vi "Scan time Input.vi"(11 "In":u32=30) -> (3 "out":u32)   [LabVIEW 2011]
doc: "ID=0x6001"
uses:
  <vilib>/Utility/miscctls.llb/LVSelectionTypeDef.ctl
panel:
  in  "cancel":bool
  in  "ok":bool
  in  "Scan Time":u32=10 caption="请输入数值:" min=1 max=10000 step=1
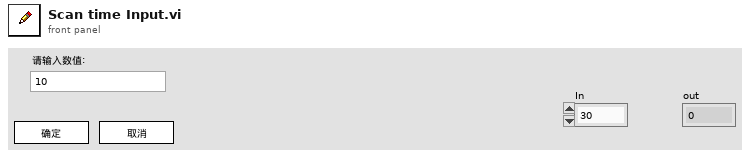
[diagram p1: front panel]
types:
  T1 = typedef "LVSelectionTypeDef.ctl" = cluster{"Selection Start":u32, "Selection End":u32}
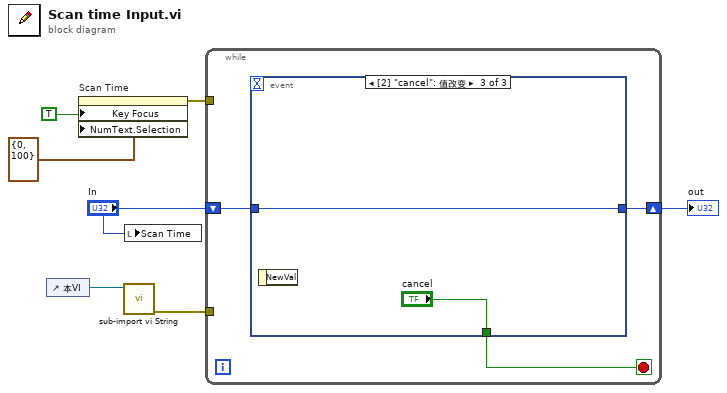
[diagram p0: block diagram]
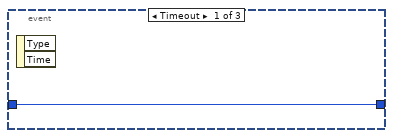
[diagram p2: hidden frame]
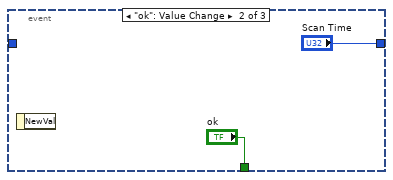
[diagram p3: hidden frame]
diagram:
  n1 = control-ref of="本VI"() -> (w2:refnum<vi>)
  n2 = property on="Scan Time" class="DigNum (严格)"("Key Focus"=TRUE ("键选中"), "NumText.Selection"=T1 {"Selection Start"=0, "Selection End"=100} ("数值文本.选择")) -> (error out=w6:errorcluster)  [unwired: 2 in, 1 out]
  n3 = call "sub-import vi String.vi"("vi ref"=w2) -> ("error out"=w1:errorcluster)  [unwired: 10 in]
  n4 = local write "Scan Time"("In") -> ()
  n5 = while {
    shift-right: [w9] -> w7
    shift-left: "In" -> [w10]
    tunnel: w6 -> [_]
    tunnel: w1 -> [_]
    stop <- w8 stop-if-true
    n6 = event shown="[2] \"cancel\": 值改变" {
      selector: _ -> [_ _ _]
      dyn-events: _ -> [_ _ _]
      timeout: _ -> [_ _ _]
      tunnel: w10 -> [w11 _ w14]
      tunnel: [w11 "Scan Time" w14] -> w9
      tunnel: [_ "ok" "cancel"] -> w8
      event Timeout {
        n7 = event-data() -> ()  [unwired: 1 in, 2 out]
      }
      event "ok": Value Change {
        n8 = event-data() -> ()  [unwired: 1 in, 1 out]
      }
      event "cancel": Value Change {
        n9 = event-data() -> ()  [unwired: 1 in, 1 out]
      }
    }
  }
  "out" <- w7
